vi "Status.vi"(8 "error in (no error)":errorcluster, 10 "data":variant, 11 "Control-Client in":refnum<class "Control-Client.lvclass">) -> (0 "error out":errorcluster, 2 "error IO":errorcluster, 3 "Control-Client out":refnum<class "Control-Client.lvclass">)   [LabVIEW 2019, in "Control-Client.lvclass"]
uses:
  Control-Client.lvclass
  dependecies/ControlsVIs/Clusters-def/CONTROL-Reply-Status-client.ctl
  dependecies/ControlsVIs/Clusters-def/DL-Reply-to-Connect-to-Client.ctl
  dependecies/ControlsVIs/Clusters-def/DAQmx-Reply-Connect-client.ctl
  dependecies/ControlsVIs/Clusters-def/OSc-Reply-Connect-client.ctl
  Delay Line/DelayLine.lvclass
  Oscilloscope/Oscilloscope.lvclass
  DAQmxTasks/DAQmxTaskContainer_General/DAQmxTaksContainer_General.lvclass
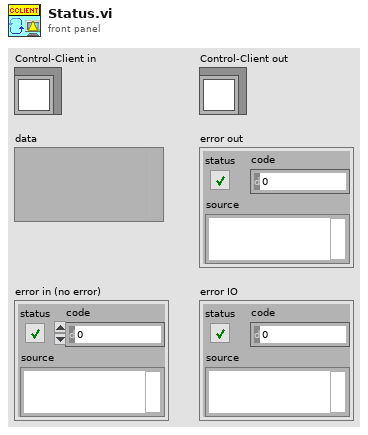
[diagram p1: front panel]
types:
  T1 = typedef "Control-Client.lvclass/CONTROL-Reply-Status-client.ctl" = cluster{"DL reply to client":T2, "Det reply to client":cluster{"on/off":bool, "calibration":dbl[], "error out":errorcluster}, "DAQmx reply to client":T3, "OSc reply to CLIENT":T4}
  T2 = typedef "DelayLine.lvclass/DL-Reply-to-Connect-to-Client.ctl" = cluster{"on/off":bool, "pos":dbl[], "param":cluster{"min":dbl, "max":dbl, "real pos":dbl}[], "predefine_pos":dbl[][], "error":errorcluster}
  T3 = typedef "DAQmxTaksContainer_General.lvclass/DAQmx-Reply-Connect-client.ctl" = cluster{"on/off":bool, "RelayKeyHeater/off":bool, "LaserShutter":bool, "AcceleratorShutter":bool, "Power":bool, "Faraday Cup Status":bool, "Pump Start_Stop":bool, "error":errorcluster}
  T4 = typedef "Oscilloscope.lvclass/OSc-Reply-Connect-client.ctl" = cluster{"on/off":bool, "WCM_state":bool, "error":errorcluster}
  T5 = cluster{"on/off":bool, "calibration":dbl[], "error out":errorcluster}
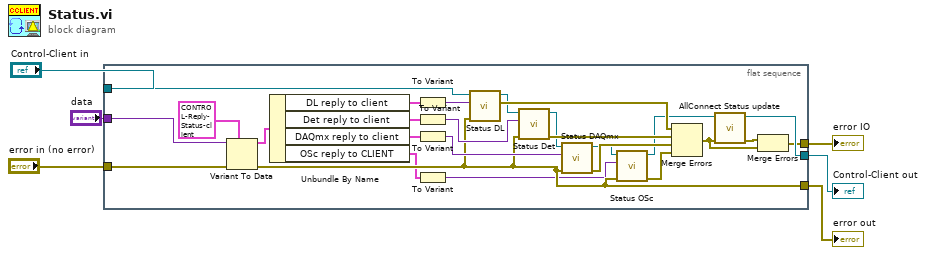
[diagram p0: block diagram]
diagram:
  n1 = flat-sequence {
    tunnel: "data" -> [w32]
    tunnel: "Control-Client in" -> [w26]
    tunnel: "error in (no error)" -> [w31]
    tunnel: [w14] -> w3
    tunnel: [w9] -> w2
    tunnel: [w17] -> w1
    frame #0 {
      n2 = Variant To Data(error in=w31, type=T1 {"DL reply to client"={"on/off"=FALSE, "pos"=[], "param"=[], "predefine_pos"=[], "error"={"status"=FALSE, "code"=0, "source"=""}}, "Det reply to client"={"on/off"=FALSE, "calibration"=[], "error out"={"status"=FALSE, "code"=0, "source"=""}}, "DAQmx reply to client"={"on/off"=FALSE, "RelayKeyHeater/off"=FALSE, "LaserShutter"=FALSE, "AcceleratorShutter"=FALSE, "Power"=FALSE, "Faraday Cup Status"=FALSE, "Pump Start_Stop"=FALSE, "error"={"status"=FALSE, "code"=0, "source"=""}}, "OSc reply to CLIENT"={"on/off"=FALSE, "WCM_state"=FALSE, "error"={"status"=FALSE, "code"=0, "source"=""}}} ("output cluster"), Variant=w32) -> (data=w29:T1, error out=w9:errorcluster)
      n3 = Unbundle By Name(w29) -> ("DL reply to client"=w27:T2, "Det reply to client"=w19:T5, "DAQmx reply to client"=w20:T3, "OSc reply to CLIENT"=w8:T4)
      n4 = To Variant(anything=w27) -> (Variant=w25:variant)
      n5 = To Variant(anything=w19) -> (Variant=w18:variant)
      n6 = To Variant(anything=w20) -> (Variant=w28:variant)
      n7 = To Variant(anything=w8) -> (Variant=w7:variant)
      n8 = call "Status DL.vi"("error in (no error)"=w9, "data"=w25, "Control-Client in"=w26) -> ("error IO"=w24:errorcluster, "Control-Client out"=w22:refnum<class "Control-Client.lvclass">)  [unwired: 6 in, 1 out]
      n9 = call "Status Det.vi"("error in (no error)"=w9, "data"=w18, "Control-Client in"=w22) -> ("error out"=w23:errorcluster, "Control-Client out"=w21:refnum<class "Control-Client.lvclass">)  [unwired: 6 in, 1 out]
      n10 = call "Status DAQmx.vi"("error in (no error)"=w9, "data"=w28, "Control-Client in"=w21) -> ("error out"=w13:errorcluster, "Control-Client out"=w11:refnum<class "Control-Client.lvclass">)  [unwired: 6 in, 1 out]
      n11 = call "Status OSc.vi"("error in (no error)"=w9, "data"=w7, "Control-Client in"=w11) -> ("error out"=w12:errorcluster, "Control-Client out"=w10:refnum<class "Control-Client.lvclass">)  [unwired: 6 in, 1 out]
      n12 = Merge Errors(w24, w23, w13, w12) -> (w15:errorcluster)
      n13 = call "AllConnect Status update.vi"("error in (no error)"=w15, "Control-Client in"=w10) -> ("error out"=w16:errorcluster, "Control-Client out"=w17:refnum<class "Control-Client.lvclass">)  [unwired: 8 in]
      n14 = Merge Errors(w16, w15) -> (w14:errorcluster)
    }
  }
  "error IO" <- w3
  "error out" <- w2
  "Control-Client out" <- w1
